vi "LocalPosition.vi"(1 "Position":T1, 2 "Total Bounds Rect":T2) -> (0 "Local Position":T1)   [LabVIEW 2014, in "Raspberry Pi Compatible Compiler for LabVIEW.lvlib" / "PythonConverter_GUI.lvclass"]
uses:
  PythonConverter_GUI.lvclass
  <vilib>/Utility/miscctls.llb/LVRectTypeDef.ctl
  <vilib>/Utility/miscctls.llb/LVPositionTypeDef.ctl
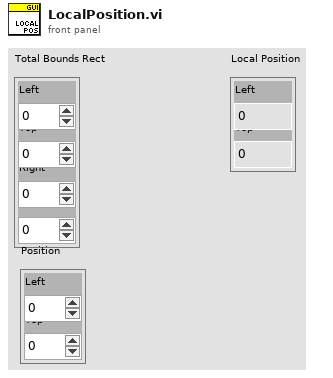
[diagram p1: front panel]
types:
  T1 = typedef "LVPositionTypeDef.ctl" = cluster{"Left":i32, "Top":i32}
  T2 = typedef "LVRectTypeDef.ctl" = cluster{"Left":i16, "Top":i16, "Right":i16, "Bottom":i16}
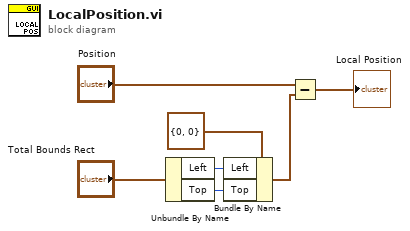
[diagram p0: block diagram]
diagram:
  n1 = Unbundle By Name("Total Bounds Rect") -> ("Left"=w5:i16, "Top"=w4:i16)
  n2 = Bundle By Name(cluster=T1 {"Left"=0, "Top"=0} ("Position"), "Left"=w5, "Top"=w4) -> (w2:T1)
  n3 = Subtract(x="Position", y=w2) -> (x-y=→"Local Position":T1)
